vi "toInstrumentScript.vi"(8 "error in (no error)":errorcluster, 11 "AnalogDevice in":refnum<class "AnalogDevice.lvclass">) -> (0 "error out":errorcluster, 2 "instrument_ScriptXml":refnum<class "xmlNode.lvclass">, 3 "AnalogDevice out":refnum<class "AnalogDevice.lvclass">)   [LabVIEW 2009, in "Tools.lvlib" / "DatabaseHelpers.lvlib" / "AnalogDevice.lvclass"]
uses:
  AnalogDevice.lvclass
  xmlNode/xmlNode.lvclass
  device.lvclass
  Scripting/ScriptingEvent/ScriptEventList/ScriptEventList.lvclass
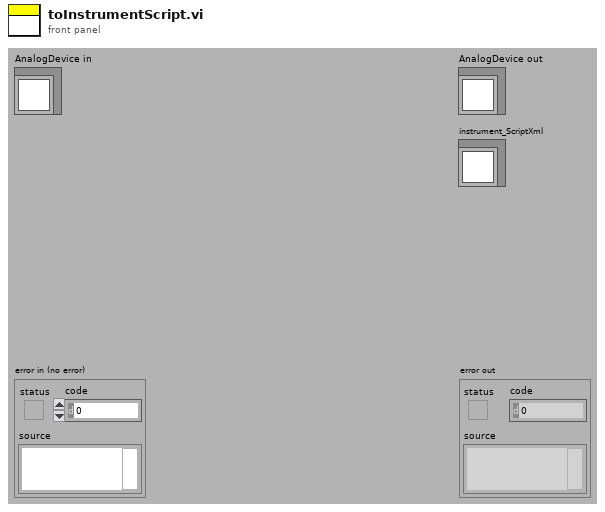
[diagram p1: front panel]
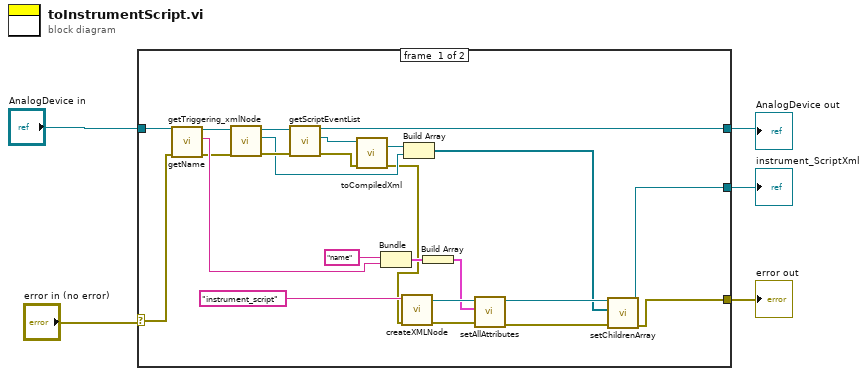
[diagram p0: block diagram]
diagram:
  n1 = case shown="No Error" "error in (no error)" {
    selector: "error in (no error)" -> [w19 w30]
    tunnel: "AnalogDevice in" -> [w20 w31]
    tunnel: [w8 w31] -> w3
    tunnel: [w21 w30] -> w2
    tunnel: [w6 _] -> w1
    frame #0 {
      n2 = call "getName.vi"("error in (no error)"=w19, "device.lvclass in"=w20) -> ("error out"=w16:errorcluster, "name"=w18:string, "device.lvclass out"=w17:refnum<class "AnalogDevice.lvclass">)  [unwired: 7 in]
      n3 = call "getTriggering_xmlNode.vi"("error in (no error)"=w16, "device.lvclass in"=w17) -> ("error out"=w14:errorcluster, "triggering_xmlNode"=w10:refnum<class "xmlNode.lvclass">, "device.lvclass out"=w15:refnum<class "AnalogDevice.lvclass">)  [unwired: 7 in]
      n4 = call "getScriptEventList.vi"("error in (no error)"=w14, "device.lvclass in"=w15) -> ("error out"=w12:errorcluster, "ScriptEventList"=w13:refnum<class "ScriptEventList.lvclass">, "device.lvclass out"=w8:refnum<class "AnalogDevice.lvclass">)  [unwired: 7 in]
      n5 = call "toCompiledXml.vi"("error in (no error)"=w12, "ScriptEventList in"=w13) -> ("error out"=w7:errorcluster, "compiledXml"=w11:refnum<class "xmlNode.lvclass">)  [unwired: 7 in, 1 out]
      n6 = Bundle("name", "name"=w18) -> (w25:cluster{string, "name":string})  [unwired: 1 in]
      n7 = call "createXMLNode.vi"("error in (no error)"=w7, "name"="instrument_script") -> ("error out"=w27:errorcluster, "xmlNode out"=w28:refnum<class "xmlNode.lvclass">)  [unwired: 8 in]
      n8 = Build Array(w11, w10) -> (w9:refnum<class "xmlNode.lvclass">[])
      n9 = Build Array(w25) -> (w24:cluster{string, "name":string}[])
      n10 = call-dynamic "setAllAttributes.vi"("error in (no error)"=w27, "attributes"=w24, "xmlNode in"=w28) -> ("error out"=w22:errorcluster, "xmlNode out"=w23:refnum<class "xmlNode.lvclass">)  [unwired: 7 in]
      n11 = call-dynamic "setChildrenArray.vi"("error in (no error)"=w22, "Children"=w9, "xmlNode.lvclass in"=w23) -> ("error out"=w21:errorcluster, "xmlNode.lvclass out"=w6:refnum<class "xmlNode.lvclass">)  [unwired: 7 in]
    }
    frame #1 {
    }
  }
  "error out" <- w2
  "AnalogDevice out" <- w3
  "instrument_ScriptXml" <- w1
